vi "Begin.vi"(8 "error in":errorcluster, 11 "COM Port":refnum<visa-resource-name>="COM4") -> (0 "error out":errorcluster)   [LabVIEW 2018]
uses:
  <vilib>/Instr/_visa.llb/VISA Configure Serial Port (Instr).vi
panel:
  out "received":string
  # "RFID INI Start"
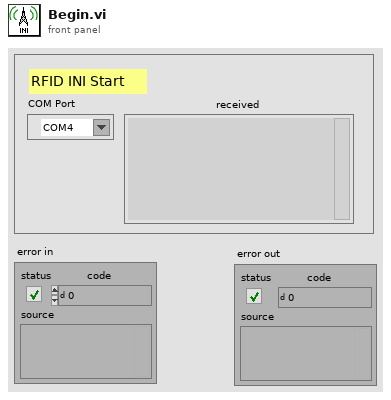
[diagram p1: front panel]
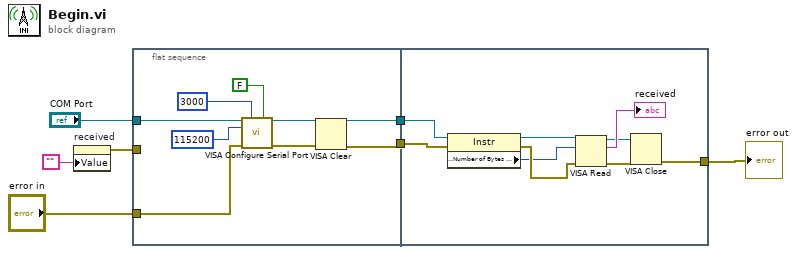
[diagram p0: block diagram]
diagram:
  n1 = property on="received" class="Str"("Value"="") -> (error out=w5:errorcluster)  [unwired: 2 in, 1 out]
  n2 = flat-sequence {
    tunnel: "COM Port" -> [w16]
    tunnel: [w8] -> w6
    tunnel: w5 -> [_]
    tunnel: "error in" -> [w12]
    tunnel: [w11] -> w1
    tunnel: w6 -> [w24]
    tunnel: [w17] -> w3
    tunnel: w1 -> [w25]
    frame #0 {
      n3 = call-poly "VISA Configure Serial Port"("VISA resource name"=w16, "timeout (10sec)"=u32 3000, "Enable Termination\nChar (T)"=FALSE ("Enable Termination\nChar (T)"), "baud rate (9600)"=u32 115200, "error in (no error)"=w12) -> ("VISA resource name out"=w10:refnum<visa-resource-name>, "error out"=w9:errorcluster)  [unwired: 9 in]
      n4 = VISA Clear(VISA resource name=w10, error in (no error)=w9) -> (VISA resource name out=w11:refnum<visa-resource-name>, error out=w8:errorcluster)
    }
    frame #1 {
      n5 = property class="Instr"(reference=w25, error in=w24) -> (reference out=w23:refnum<visa-resource-name>, error out=w22:errorcluster, "Serial Settings:Number of Bytes at Serial Port"=w21:u32)
      n6 = VISA Read(VISA resource name=w23, byte count=w21, error in (no error)=w22) -> (VISA resource name out=w19:refnum<visa-resource-name>, read buffer=→"received":string, error out=w18:errorcluster)  [unwired: 1 out]
      n7 = VISA Close(VISA resource name=w19, error in (no error)=w18) -> (error out=w17:errorcluster)
    }
  }
  "error out" <- w3
